vi "Write loopCounter.vi"(8 "error in (no error)":errorcluster, 10 "loopCounter":i32, 11 "ExampleTask_StopNotifier in":refnum<class "Task_BoolStopNotifier.lvclass">) -> (0 "error out":errorcluster, 3 "ExampleTask_StopNotifier out":refnum<class "Task_BoolStopNotifier.lvclass">)   [LabVIEW 2023, in "Task_BoolStopNotifier.lvclass"]
doc: "_____________________________________\nTLC Daemon 1.0.0.2\nCopyright (c) 2026 Andrea Cadei"
uses:
  Task_BoolStopNotifier.lvclass
  Task_BoolStopNotifier.lvclass/Task_BoolStopNotifier.ctl
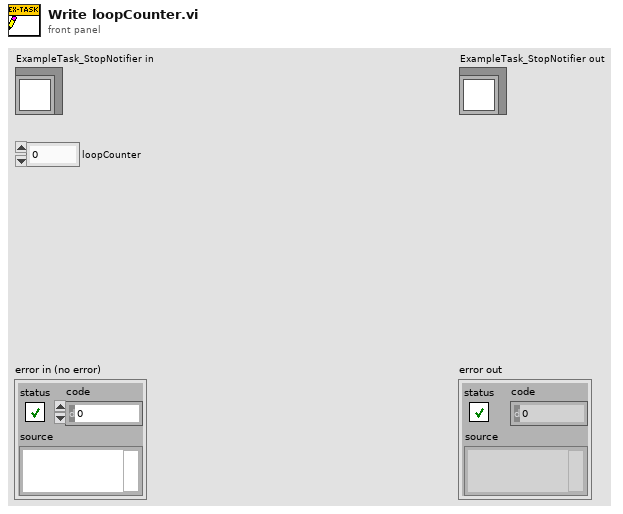
[diagram p1: front panel]
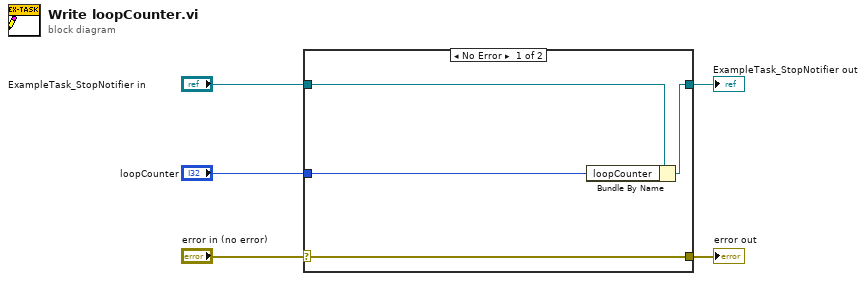
[diagram p0: block diagram]
diagram:
  n1 = case shown="No Error" "error in (no error)" {
    selector: "error in (no error)" -> [w9 w10]
    tunnel: [w9 w10] -> w4
    tunnel: [w7 w11] -> w2
    tunnel: "ExampleTask_StopNotifier in" -> [w8 w11]
    tunnel: "loopCounter" -> [w6 _]
    frame No Error {
      n2 = Bundle By Name(cluster=w8, "loopCounter"=w6) -> (w7:refnum<class "Task_BoolStopNotifier.lvclass">)
    }
    frame Error {
    }
  }
  "error out" <- w4
  "ExampleTask_StopNotifier out" <- w2
